vi "Create Custom Device.vi"(8 "error in (no error)":errorcluster, 9 "J1939 Monitor Settings":T2 {"Name" format="%.0x"}, 10 "J1939 XNET Settings":T3 {"Termination" items=["Off", "On"]}, 11 "Device Item Ref in":T1 format="%.0x") -> (0 "error out":errorcluster, 2 "Monitor Ref out":T1 format="%.0x", 3 "Device Item Ref out":T1 format="%.0x")   [LabVIEW 2023, in "J1939 System Definition API Support.lvlib"]
uses:
  J1939 System Definition API Support.lvlib
  Addon/Addon Shared/Types/XNET Settings.ctl
  Addon/Addon Shared/Types/Monitor Settings.ctl
  <vilib>/NI VeriStand/Custom Device API/Custom Device Item Ref.ctl
  Addon/Addon Shared/J1939 Addon Shared.lvlib
  <vilib>/NI VeriStand/Custom Device API/Custom Device API.lvlib
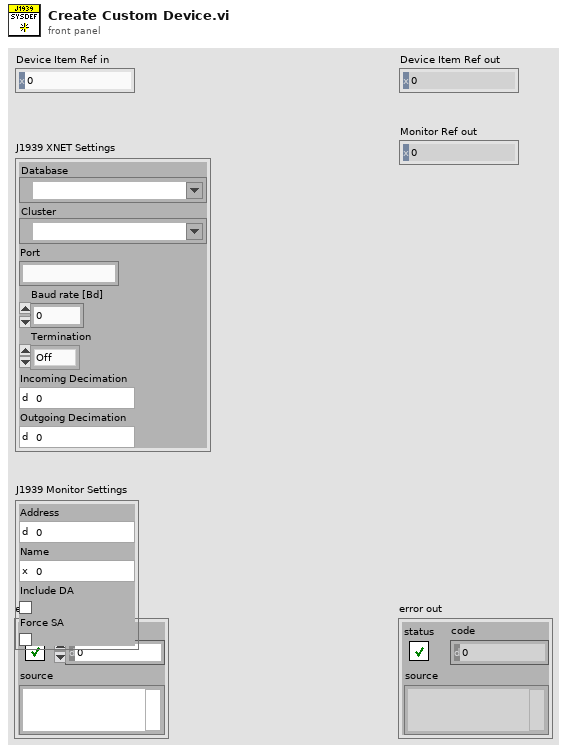
[diagram p1: front panel]
types:
  T1 = typedef "Custom Device API.lvlib/Custom Device Item Ref.ctl" = u64
  T2 = typedef "J1939 Addon Shared.lvlib/Monitor Settings.ctl" = cluster{"Address":u8, "Name":u64, "Include DA":bool, "Force SA":bool}
  T3 = typedef "J1939 Addon Shared.lvlib/XNET Settings.ctl" = cluster{"Database":refnum<k21>, "Cluster":refnum<k21>, "Port":string, "Baud rate [Bd]":u32, "Termination":u32, "Incoming Decimation":u32, "Outgoing Decimation":u32}
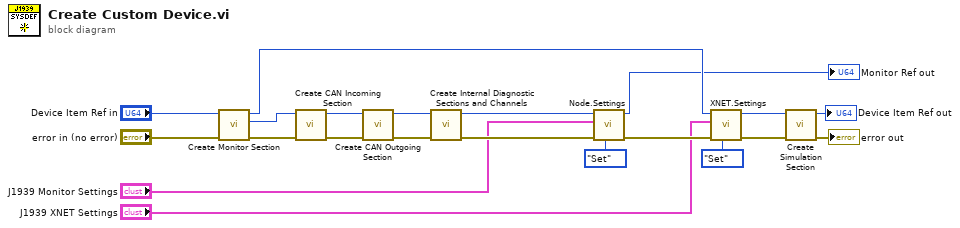
[diagram p0: block diagram]
diagram:
  n1 = call "Create Monitor Section.vi"("error in (no error)"="error in (no error)", "Device Item Ref in"="Device Item Ref in") -> ("error out"=w17:errorcluster, "Section Ptr"=w16:T1, "Parent Ref out"=w13:T1)  [unwired: 7 in]
  n2 = call "Create CAN Incoming Section.vi"("error in (no error)"=w17, "Device Item Ref in"=w16) -> ("error out"=w18:errorcluster, "Device Item Ref Out"=w19:T1)  [unwired: 8 in]
  n3 = call "Create CAN Outgoing Section.vi"("error in (no error)"=w18, "Parent Ref in"=w19) -> ("error out"=w21:errorcluster, "Parent Ref out"=w20:T1)  [unwired: 8 in]
  n4 = call "Create Internal Diagnostic Sections and Channels.vi"("error in (no error)"=w21, "Device Item Ref in"=w20) -> ("error out"=w11:errorcluster, "Device Item Ref Out"=w9:T1)  [unwired: 8 in]
  n5 = call "Node.Settings.vi"("Action"=enum8{"Get", "Set"}."Set", "error in (no error)"=w11, "Node.Settings"="J1939 Monitor Settings", "Item Ref in"=w9) -> ("error out"=w10:errorcluster, "Item Ref out"=→"Monitor Ref out":T1)  [unwired: 5 in, 1 out]
  n6 = call "XNET.Settings.vi"("Action"=enum8{"Get", "Set"}."Set", "error in (no error)"=w10, "J1939 XNET Settings"="J1939 XNET Settings", "Parent Ref in"=w13) -> ("error out"=w15:errorcluster, "Item Ref out"=w12:T1)  [unwired: 5 in, 1 out]
  n7 = call "Create Simulation Section.vi"("error in (no error)"=w15, "Parent Ref in"=w12) -> ("error out"=→"error out":errorcluster, "Parent Ref out"=→"Device Item Ref out":T1)  [unwired: 7 in, 1 out]
